vi "kdtree.vi"(7 "depth_max":i32=7, 11 "in":dbl[][](array[numeric])) -> (0 "time":u32, 3 "out":dbl[][](array[numeric]))   [LabVIEW 2012]
panel:
  out "size(s)":i32[](array[numeric])
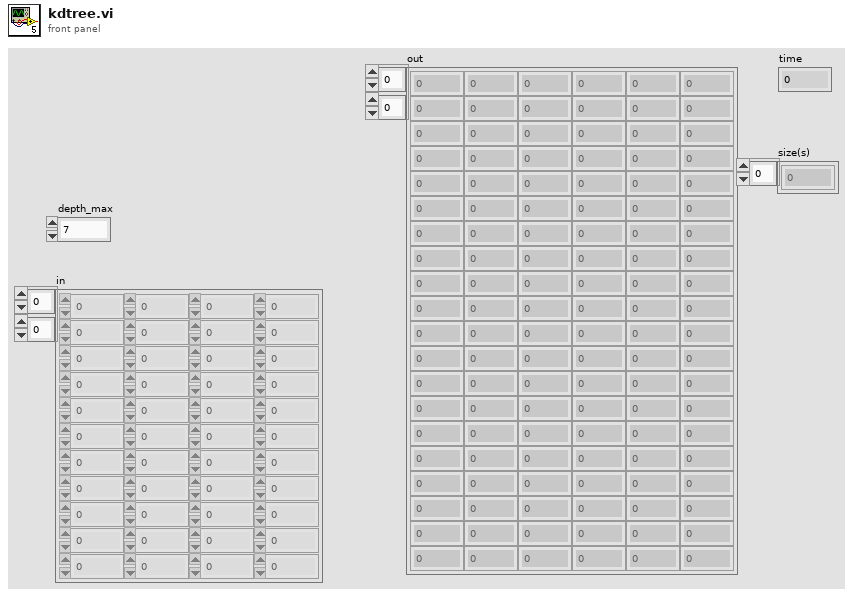
[diagram p1: front panel]
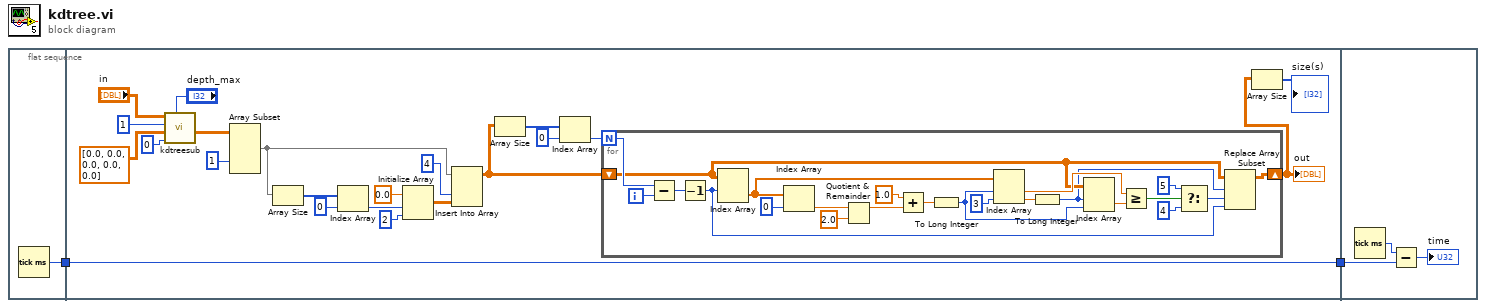
[diagram p0: block diagram]
diagram:
  n1 = flat-sequence {
    tunnel: [w3] -> w2
    tunnel: w2 -> [w7]
    tunnel: [w7] -> w1
    tunnel: w1 -> [w50]
    frame #0 {
      n2 = Tick Count (ms)() -> (millisecond timer value=w3:u32)
    }
    frame #1 {
      n3 = call "kdtreesub.vi"("depth_max"="depth_max", "mom"=0, "out"=dbl[][] [[0.0, 0.0, 0.0, 0.0, 0.0]], "depth"=1, "in"="in") -> ("out 2"=w20:dbl[][])  [unwired: 6 in]
      n4 = Array Subset(array=w20, index (col)=1 ("index")) -> (w13:dbl[][])  [unwired: 3 in]
      n5 = Array Size(array=w13) -> (size(s)=w18:i32[])
      n6 = Index Array(array=w18, index=0) -> (element=w16:i32)
      n7 = Initialize Array(0.0 ("element"), w16, 2 ("dimension size")) -> (w11:dbl[][])
      n8 = Insert Into Array(array=w13, index (col)=4 ("disabled index (col)"), new element=w11) -> (w25:dbl[][])  [unwired: 1 in]
      n9 = Array Size(array=w25) -> (size(s)=w10:i32[])
      n10 = Index Array(array=w10, index=0) -> (element=w8:i32)
      n11 = for {
        N: w8 -> [w48]
        shift-right: [w31] -> w5
        shift-left: w25 -> [w33]
        i -> [w47]
        n12 = Subtract(x=w48, y=w47) -> (x-y=w46:i32)
        n13 = Decrement(x=w46) -> (x-1=w32:i32)
        n14 = Index Array(array=w33, index (row)=w32) -> (element=w40:dbl[])  [unwired: 1 in]
        n15 = Index Array(array=w40, index=0) -> (element=w44:dbl)
        n16 = Quotient & Remainder(x=w44, y=2.0) -> (x-y*floor(x/y)=w42:dbl)  [unwired: 1 out]
        n17 = Add(x=1.0, y=w42) -> (x+y=w39:dbl)
        n18 = To Long Integer(number=w39) -> (32bit integer=w36:i32)
        n19 = Index Array(array=w40, index #1=w36, index #2=3 ("index")) -> (element #1=w34:dbl, element #2=w37:dbl)
        n20 = To Long Integer(number=w37) -> (32bit integer=w26:i32)
        n21 = Index Array(array=w33, index (row)=w26, index (col)=w36) -> (element=w35:dbl)
        n22 = Greater Or Equal?(x=w34, y=w35) -> (x >= y?=w30:bool)
        n23 = Select(t=5 ("disabled index (col)"), s=w30, f=4 ("disabled index (col)")) -> (s? t:f=w29:i32)
        n24 = Replace Array Subset(array=w33, new element=w32, index (row)=w26, index (col)=w29) -> (w31:dbl[][])
      }
      "out" <- w5
      n25 = Array Size(array=w5) -> (size(s)=→"size(s)":i32[])
    }
    frame #2 {
      n26 = Tick Count (ms)() -> (millisecond timer value=w51:u32)
      n27 = Subtract(x=w51, y=w50) -> (x-y=→"time":u32)
    }
  }
